vi "ConfigureOutput.vi"(8 "error in (no error)":errorcluster, 10 "Output((F)":bool, 11 "YP03-60_X in":refnum<class "YP03-60_X.lvclass">) -> (0 "error out 2":errorcluster, 3 "YP03-60_X out":refnum<class "YP03-60_X.lvclass">)   [LabVIEW 2020, in "PowerControl.lvlib" / "YP03-60_X.lvclass"]
uses:
  YP03-60_X.lvclass
  YP03-60_X.lvclass/YP03-60_X.ctl
  <vilib>/Instr/_visa.llb/VISA Configure Serial Port (Instr).vi
  VirtualPower/VirtualPower.lvclass
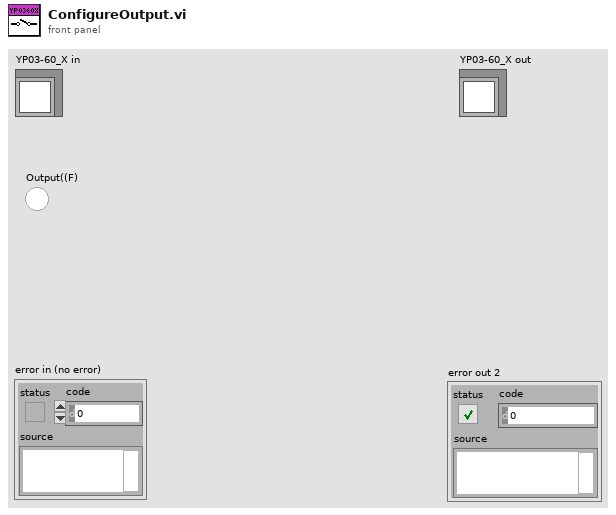
[diagram p1: front panel]
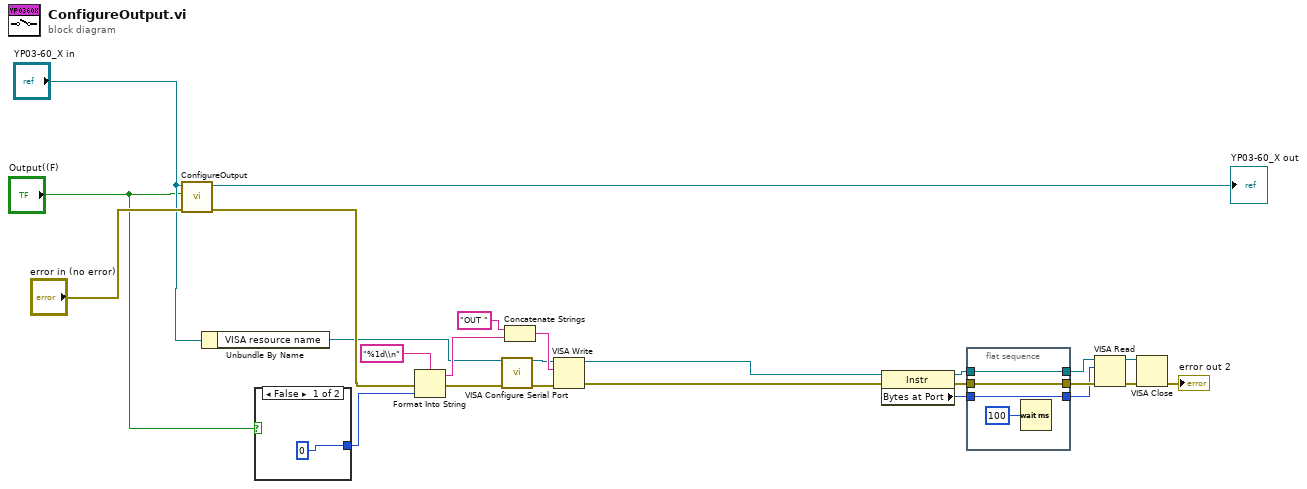
[diagram p0: block diagram]
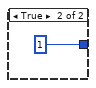
[diagram p2: hidden frame]
diagram:
  n1 = call-parent "ConfigureOutput.vi"("error in (no error)"="error in (no error)", "Output((F)"="Output((F)", "VirtualPower in"="YP03-60_X in") -> ("error out"=w10:errorcluster, "VirtualPower out"=→"YP03-60_X out":refnum<class "YP03-60_X.lvclass">)  [unwired: 7 in]
  n2 = Unbundle By Name("YP03-60_X in") -> ("VISA resource name"=w5:refnum<visa-resource-name>)
  n3 = case shown="False" "Output((F)" {
    tunnel: [0 1] -> w1
    frame False {
    }
    frame True {
    }
  }
  n4 = Format Into String(format string="%1d\\n", error in=w10, w1) -> (resulting string=w13:string, error out=w8:errorcluster)  [unwired: 1 in]
  n5 = call-poly "VISA Configure Serial Port"("VISA resource name"=w5, "error in (no error)"=w8) -> ("VISA resource name out"=w6:refnum<visa-resource-name>, "error out"=w7:errorcluster)  [unwired: 12 in]
  n6 = Concatenate Strings("OUT " ("string"), w13) -> (w16:string)
  n7 = VISA Write(VISA resource name=w6, write buffer=w16, error in (no error)=w7) -> (VISA resource name out=w14:refnum<visa-resource-name>, error out=w15:errorcluster)  [unwired: 1 out]
  n8 = property class="Instr"(reference=w14, error in=w15) -> (reference out=w19:refnum<visa-resource-name>, error out=w21:errorcluster, "Bytes at Port"=w17:u32)
  n9 = flat-sequence {
    tunnel: w19 -> [w31]
    tunnel: [w31] -> w20
    tunnel: [w30] -> w22
    tunnel: w21 -> [w30]
    tunnel: [w29] -> w18
    tunnel: w17 -> [w29]
    frame #0 {
      n10 = Wait (ms)(milliseconds to wait=u32 100) -> ()  [unwired: 1 out]
    }
  }
  n11 = VISA Read(VISA resource name=w20, byte count=w18, error in (no error)=w22) -> (VISA resource name out=w2:refnum<visa-resource-name>, error out=w4:errorcluster)  [unwired: 2 out]
  n12 = VISA Close(VISA resource name=w2, error in (no error)=w4) -> (error out=→"error out 2":errorcluster)
